vi "Chassis_Sensors.vi"() -> ()   [LabVIEW 2018]
uses:
  Global Variables.vi
panel:
  out "SubVi Info":T1(array[cluster])
  in  "?":T2={"Sample Rate"=1000.0, "samples per channel"=100, "DAQmx Device Name"="Current_PXI_1"}
  in  "?":T2={"Sample Rate"=90.0, "samples per channel"=100, "DAQmx Device Name"="TC_PXI_1"}
  in  "?":T2={"Sample Rate"=90.0, "samples per channel"=9, "DAQmx Device Name"=""}
  in  "Alicat_O2":T3={"O2 [ A-19200-COM17]"={" ID"="A", "Baud "=enum."19200", "VISA Sesssion In"="COM17"}}
  in  "Alicat_Ar":T4={"AR [ B-19200-COM14]"={" ID"="B", "Baud "=enum."19200", "VISA Sesssion In"="COM14"}}
  in  "Use Sensor?":bool=TRUE
  in  "Use Sensor?":bool=TRUE
  in  "Use Sensor?":bool
  in  "Use Sensor?":bool=TRUE
  in  "Use Sensor?":bool=TRUE
  in  "Ring":u16(ring)=1 items=["Alicat", "DAQmx"]
  in  "stop":bool
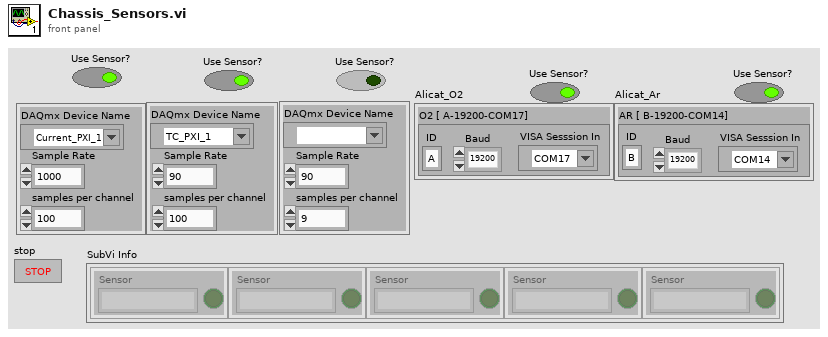
[diagram p1: front panel]
types:
  T1 = cluster{"Sensor":string, "Panel Ref Out":refnum<vi>, bool}[]
  T2 = cluster{"Sample Rate":dbl, "samples per channel":i32, "DAQmx Device Name":tag}
  T3 = cluster{"O2 [ A-19200-COM17]":cluster{" ID":string, "Baud ":enum8{"2400", "9600", "19200", "38400", "57600", "115200", "Unknown"}, "VISA Sesssion In":refnum<visa-resource-name>}}
  T4 = cluster{"AR [ B-19200-COM14]":cluster{" ID":string, "Baud ":enum8{"2400", "9600", "19200", "38400", "57600", "115200", "Unknown"}, "VISA Sesssion In":refnum<visa-resource-name>}}
  T5 = enum32{"Invalid", "Standard", "Closed", "Hidden", "Minimized", "Maximized"}
  T6 = cluster{"type":string, "Panel Ref Out":refnum<vi>, bool}
  T7 = enum32{"Bad", "Idle", "Run top level", "Running"}
  T8 = cluster{"task/channels in":string, "Panel Ref Out":refnum<vi>, bool}[]
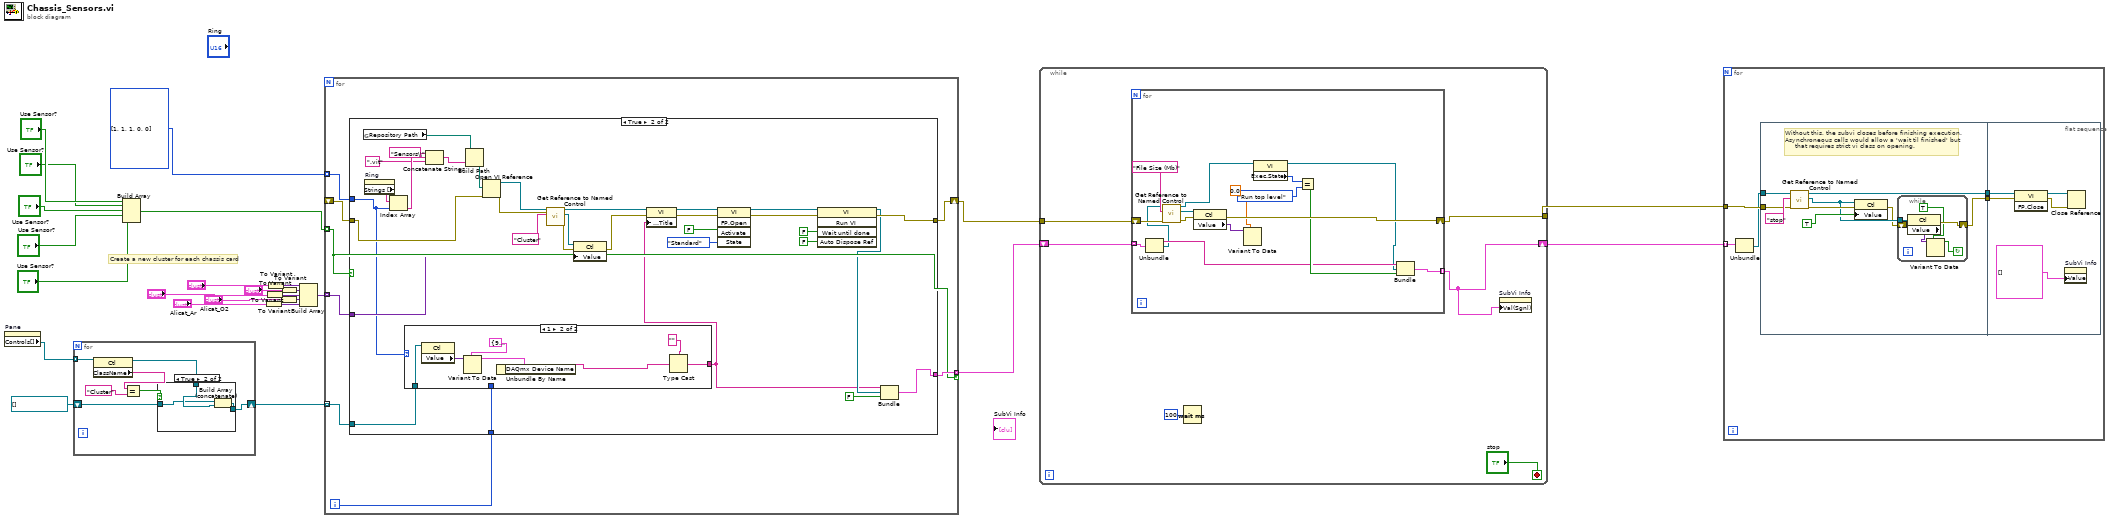
[diagram p0: block diagram]
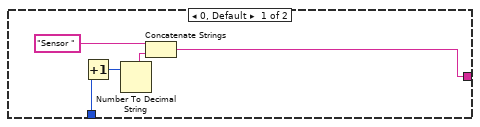
[diagram p4: hidden frame]
diagram:
  w13 = u16[] [1, 1, 1, 0, 0] items=["Alicat", "DAQmx"] ("Array 2")
  # "Create a new cluster for each chassis card"
  n1 = property on="Pane" class="Pane"() -> ("Controls[]"=w11:refnum<vi>[])  [unwired: 2 in, 2 out]
  n2 = for {
    tunnel: w11 -> [w32] mode=indexing
    shift-right: [w27] -> w9
    shift-left: refnum<vi>[] [] -> [w26]
    n3 = property class="Ctl"(reference=w32) -> (reference out=w28:refnum<vi>, "ClassName"=w29:string)  [unwired: 1 in, 1 out]
    n4 = Equal?(x=w29, y="Cluster") -> (x = y?=w31:bool)
    n5 = case shown="True" w31 {
      tunnel: w28 -> [_ w35]
      tunnel: [w33 w36] -> w27
      tunnel: w26 -> [w33 w34]
      frame False {
      }
      frame True {
        n6 = Build Array (concatenate)(w34, w35) -> (w36:refnum<vi>[])
      }
    }
  }
  n7 = Build Array("Use Sensor?", "Use Sensor?", "Use Sensor?", "Use Sensor?", "Use Sensor?") -> (w3:bool[])
  n8 = To Variant(anything="Alicat_Ar") -> (Variant=w14:variant)
  n9 = To Variant(anything="?") -> (Variant=w16:variant)
  n10 = To Variant(anything="?") -> (Variant=w18:variant)
  n11 = To Variant(anything="Alicat_O2") -> (Variant=w15:variant)
  n12 = To Variant(anything="?") -> (Variant=w17:variant)
  n13 = Build Array(w18, w17, w16, w15, w14) -> (w12:variant[])
  n14 = for {
    tunnel: w13 -> [w43] mode=indexing
    tunnel: w12 -> [w42] mode=indexing
    tunnel: w9 -> [w40] mode=indexing
    tunnel: w3 -> [w38] mode=indexing
    shift-right: [w44] -> w25
    shift-left: _ -> [w39]
    tunnel: [w41] -> w2 mode=indexing if=w38
    i -> [w37]
    n15 = case shown="True" w38 {
      tunnel: [w45 w69] -> w44
      tunnel: w43 -> [_ w55]
      tunnel: w42 -> [_ w61]
      tunnel: [_ w57] -> w41
      tunnel: w40 -> [_ w56]
      tunnel: w39 -> [w45 w59]
      tunnel: w37 -> [_ w54]
      frame False {
      }
      frame True {
        n16 = global read "Global Variables.vi" "Repository Path"() -> (w77:path)
        n17 = property on="Ring" class="Ring (strict)"() -> ("Strings []"=w66:string[])  [unwired: 2 in, 2 out]
        n18 = Index Array(array=w66, index=w55) -> (element=w63:string)
        n19 = case shown="1" w55 {
          tunnel: w56 -> [_ w86]
          tunnel: [w79 w85] -> w47
          tunnel: w54 -> [w82 _]
          frame 0, Default {
            n20 = Increment(x=w82) -> (x+1=w78:i32)
            n21 = Number To Decimal String(number=w78) -> (decimal integer string=w80:string)  [unwired: 1 in]
            n22 = Concatenate Strings("Sensor ", w80) -> (w79:string)
          }
          frame 1 {
            n23 = property class="Ctl"(reference=w86) -> ("Value"=w89:variant)  [unwired: 1 in, 2 out]
            n24 = Variant To Data(type=T2 {"Sample Rate"=90.0, "samples per channel"=9, "DAQmx Device Name"=""}, Variant=w89) -> (data=w88:T2)  [unwired: 1 in, 1 out]
            n25 = Unbundle By Name(w88) -> ("DAQmx Device Name"=w83:tag)
            n26 = Type Cast(type="", x=w83) -> (*(type *) &x=w85:string)
          }
        }
        n27 = Concatenate Strings("Sensors\\" ("string"), w63, ".vit" ("string")) -> (w65:string)
        n28 = Build Path(base path=w77, name or relative path=w65) -> (appended path=w46:path)
        n29 = Open VI Reference(vi path=w46, error in (no error)=w59) -> (vi reference=w71:refnum<vi>, error out=w70:errorcluster)  [unwired: 4 in]
        n30 = call "Get Reference to Named Control.vi"("error in (no error)"=w70, "Control Name"="Cluster" ("element"), "Front Panel Ref"=w71) -> ("error out"=w74:errorcluster, "Ctl Refnum"=w75:refnum<vi>, "Panel Ref Out"=w53:refnum<vi>)  [unwired: 6 in]
        n31 = property class="Ctl"(reference=w75, error in=w74, "Value"=w61) -> (error out=w51:errorcluster)  [unwired: 1 out]
        n32 = property class="VI"(reference=w53, error in=w51, "Front Panel.Title"=w47) -> (reference out=w52:refnum<vi>, error out=w50:errorcluster)
        n33 = invoke class="VI" method="FP.Open"(reference=w52, error in=w50, "Activate"=FALSE ("Wait Until Done"), "State"=T5."Standard") -> (reference out=w48:refnum<vi>, error out=w49:errorcluster)  [unwired: 1 in, 3 out]
        n34 = invoke class="VI" method="Run VI"(reference=w48, error in=w49, "Wait until done"=FALSE ("Wait Until Done"), "Auto Dispose Ref"=FALSE ("Auto Dispose Reference")) -> (reference out=w58:refnum<vi>, error out=w69:errorcluster)  [unwired: 1 in, 3 out]
        n35 = Bundle("type"=w47, "Panel Ref Out"=w58, FALSE) -> (w57:T6)  [unwired: 1 in]
      }
    }
  }
  n36 = while {
    tunnel: w25 -> [w95]
    tunnel: [w93] -> w24
    shift-right: [w90] -> w1
    shift-left: w2 -> [w92]
    stop <- "stop" stop-if-true
    n37 = for {
      shift-right: [w109] -> w93
      shift-left: w95 -> [w108]
      tunnel: [w101] -> w90 mode=indexing
      tunnel: w92 -> [w100] mode=indexing
      n38 = Unbundle(w100) -> ("type"=w99:string, "Panel Ref Out"=w98:refnum<vi>)  [unwired: 1 out]
      n39 = call "Get Reference to Named Control.vi"("error in (no error)"=w108, "Control Name"="File Size (Mb)" ("element"), "Front Panel Ref"=w98) -> ("error out"=w107:errorcluster, "Ctl Refnum"=w111:refnum<vi>, "Panel Ref Out"=w97:refnum<vi>)  [unwired: 6 in]
      n40 = property class="Ctl"(reference=w111, error in=w107) -> (error out=w109:errorcluster, "Value"=w106:variant)  [unwired: 1 out]
      n41 = Variant To Data(type=0.0, Variant=w106) -> ()  [unwired: 1 in, 2 out]
      n42 = property class="VI"(reference=w97) -> (reference out=w96:refnum<vi>, "Exec.State"=w104:T7)  [unwired: 1 in, 1 out]
      n43 = Equal?(x=w104, y=T7."Run top level" ("Execution:State 2")) -> (x = y?=w102:bool)
      n44 = Bundle("type"=w99, "Panel Ref Out"=w96, w102) -> (w101:T6)  [unwired: 1 in]
    }
    n45 = Wait (ms)(milliseconds to wait=u32 100) -> ()  [unwired: 1 out]
    n46 = property on="SubVi Info" class="Arr (strict)"("Val(Sgnl)"=w90) -> ()  [unwired: 2 in, 2 out]
  }
  n47 = for {
    tunnel: w24 -> [w116]
    tunnel: w1 -> [w113] mode=indexing
    n48 = Unbundle(w113) -> ("Panel Ref Out"=w112:refnum<vi>)  [unwired: 2 out]
    n49 = flat-sequence {
      tunnel: w116 -> [w124]
      tunnel: [w121] -> w115
      tunnel: [w118] -> w114
      tunnel: w112 -> [w120]
      tunnel: w115 -> [w136]
      tunnel: w114 -> [w134]
      frame #0 {
        # "Without this, the subvi closes before finishing execution.\nAsynchroneous calls would allow a 'wait til finished' but \n     that requires strict vi class on opening."
        n50 = call "Get Reference to Named Control.vi"("error in (no error)"=w124, "Control Name"="stop", "Front Panel Ref"=w120) -> ("error out"=w122:errorcluster, "Ctl Refnum"=w119:refnum<vi>, "Panel Ref Out"=w121:refnum<vi>)  [unwired: 6 in]
        n51 = property class="Ctl"(reference=w119, error in=w122, "Value"=TRUE) -> (error out=w117:errorcluster)  [unwired: 1 out]
        n52 = while {
          tunnel: w119 -> [w129]
          shift-right: [w130] -> w118
          shift-left: w117 -> [w131]
          stop <- w126 continue-if-true
          n53 = property class="Ctl"(reference=w129, error in=w131) -> (error out=w130:errorcluster, "Value"=w128:variant)  [unwired: 1 out]
          n54 = Variant To Data(type=TRUE, Variant=w128) -> (data=w126:bool)  [unwired: 1 in, 1 out]
        }
      }
      frame #1 {
        n55 = invoke class="VI" method="FP.Close"(reference=w136, error in=w134) -> (reference out=w135:refnum<vi>, error out=w133:errorcluster)  [unwired: 1 in, 1 out]
        n56 = property on="SubVi Info" class="Arr (strict)"("Value"=T8 [] ("SubVi Info")) -> ()  [unwired: 2 in, 2 out]
        n57 = Close Reference(reference=w135, error in (no error)=w133) -> ()  [unwired: 1 out]
      }
    }
  }
